vi "Get Diode Temperature.vi"(9 "Config":T1={"Channel Index"=1, "Diode TC (mV)"=1.3, "Channel name"="Source-Current", "Ref voltage"=0.8, "Ref temp"=25.0, "Gain"=25.0} {"Gain" format="%.3f"; "Ref temp" format="%.3f"; "Ref voltage" format="%.3f"; "Diode TC (mV)" format="%.3f"}, 11 "array":waveform(dbl)[](array[waveform])) -> (1 "Channel name":string, 3 "waveform out":waveform(dbl))   [LabVIEW 2019]
doc: "This example demonstrates how to acquire a continuous amount of data (Waveform) using the DAQ device's internal clock. It also shows how to synchronize two devices for different device families (E Series, S Series, M Series, X Series, DSA, and SC Express), to simultaneously acquire the data.\n\nFor instructions on how to connect your signals to the DAQ device, refer to your device documentation."
panel:
  # "Get Temperature - Diode"
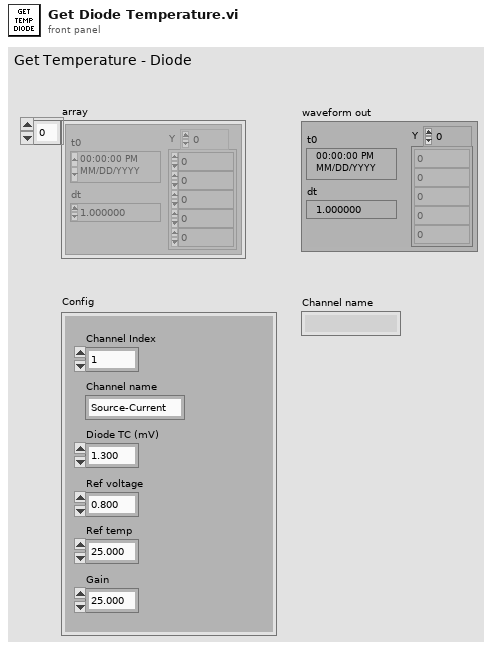
[diagram p1: front panel]
types:
  T1 = cluster{"Channel Index":i32, "Diode TC (mV)":dbl, "Channel name":string, "Ref voltage":dbl, "Ref temp":dbl, "Gain":dbl}
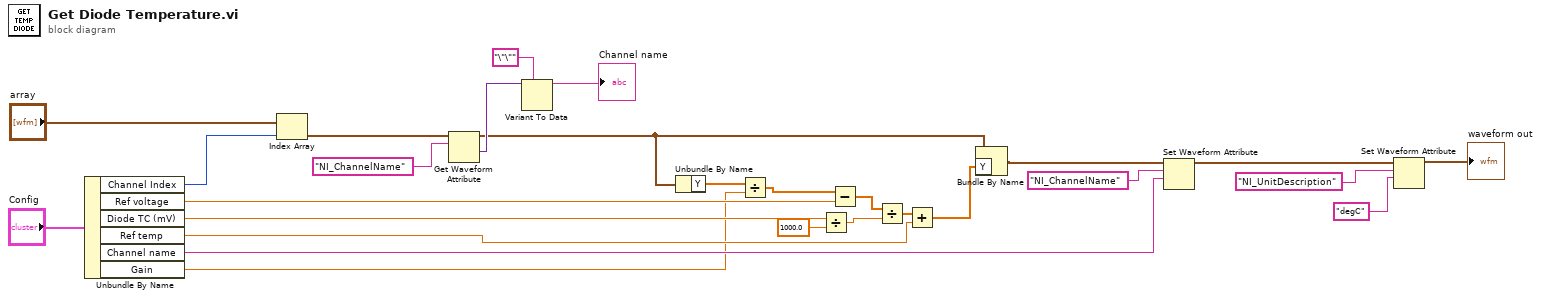
[diagram p0: block diagram]
diagram:
  n1 = Unbundle By Name("Config") -> ("Channel Index"=w18:i32, "Ref voltage"=w13:dbl, "Diode TC (mV)"=w12:dbl, "Ref temp"=w5:dbl, "Channel name"=w4:string, "Gain"=w1:dbl)
  n2 = Index Array(array="array", index=w18) -> (element=w22:waveform(dbl))
  n3 = Get Waveform Attribute(6:"NI_ChannelName" ("name"), 7:w22) -> (1:w16:variant, 3:w7:waveform(dbl))  [unwired: 2 in, 2 out]
  n4 = Variant To Data(type="\"\"" ("name"), Variant=w16) -> (data=→"Channel name":string)  [unwired: 1 in, 1 out]
  n5 = Unbundle By Name(w7) -> ("Y"=w3:dbl[])
  n6 = Divide(x=w3, y=w1) -> (x/y=w2:dbl[])
  n7 = Divide(x=w12, y=1000.0) -> (x/y=w11:dbl)
  n8 = Subtract(x=w2, y=w13) -> (x-y=w14:dbl[])
  n9 = Divide(x=w14, y=w11) -> (x/y=w9:dbl[])
  n10 = Add(x=w9, y=w5) -> (x+y=w8:dbl[])
  n11 = Bundle By Name(cluster=w7, "Y"=w8) -> (w6:waveform(dbl))
  n12 = Set Waveform Attribute(5:w4, 6:"NI_ChannelName" ("name"), 7:w6) -> (3:w24:waveform(dbl))  [unwired: 1 in, 2 out]
  n13 = Set Waveform Attribute(5:"degC" ("name"), 6:"NI_UnitDescription" ("name"), 7:w24) -> (3:→"waveform out":waveform(dbl))  [unwired: 1 in, 2 out]
